vi "Autonomous Independent.vi"   [LabVIEW 2017]
doc: "This VI is called when autonomous begins, and will automatically be terminated when autonomous ends. You can carry out timed or sensor driven robot movement independently without needing to return to the caller."
uses:
  <vilib>/Rock Robotics/WPI/ThirdParty/Sensors/navX/_TypeDefs/FRIC_navX_DeviceNumbersTypeDef.ctl
  <vilib>/Rock Robotics/Network Tables/NT Read String.vi
  Robot Global Data.vi
panel:
  # "Be sure to right-click and choose Data Operations>>Make Current Value default if you want to save the array values with the VI"
types:
  T1 = typedef "FRIC_navX_DeviceNumbersTypeDef.ctl" = enum16{"Dev0", "Dev1", "Dev2", "Dev3"}
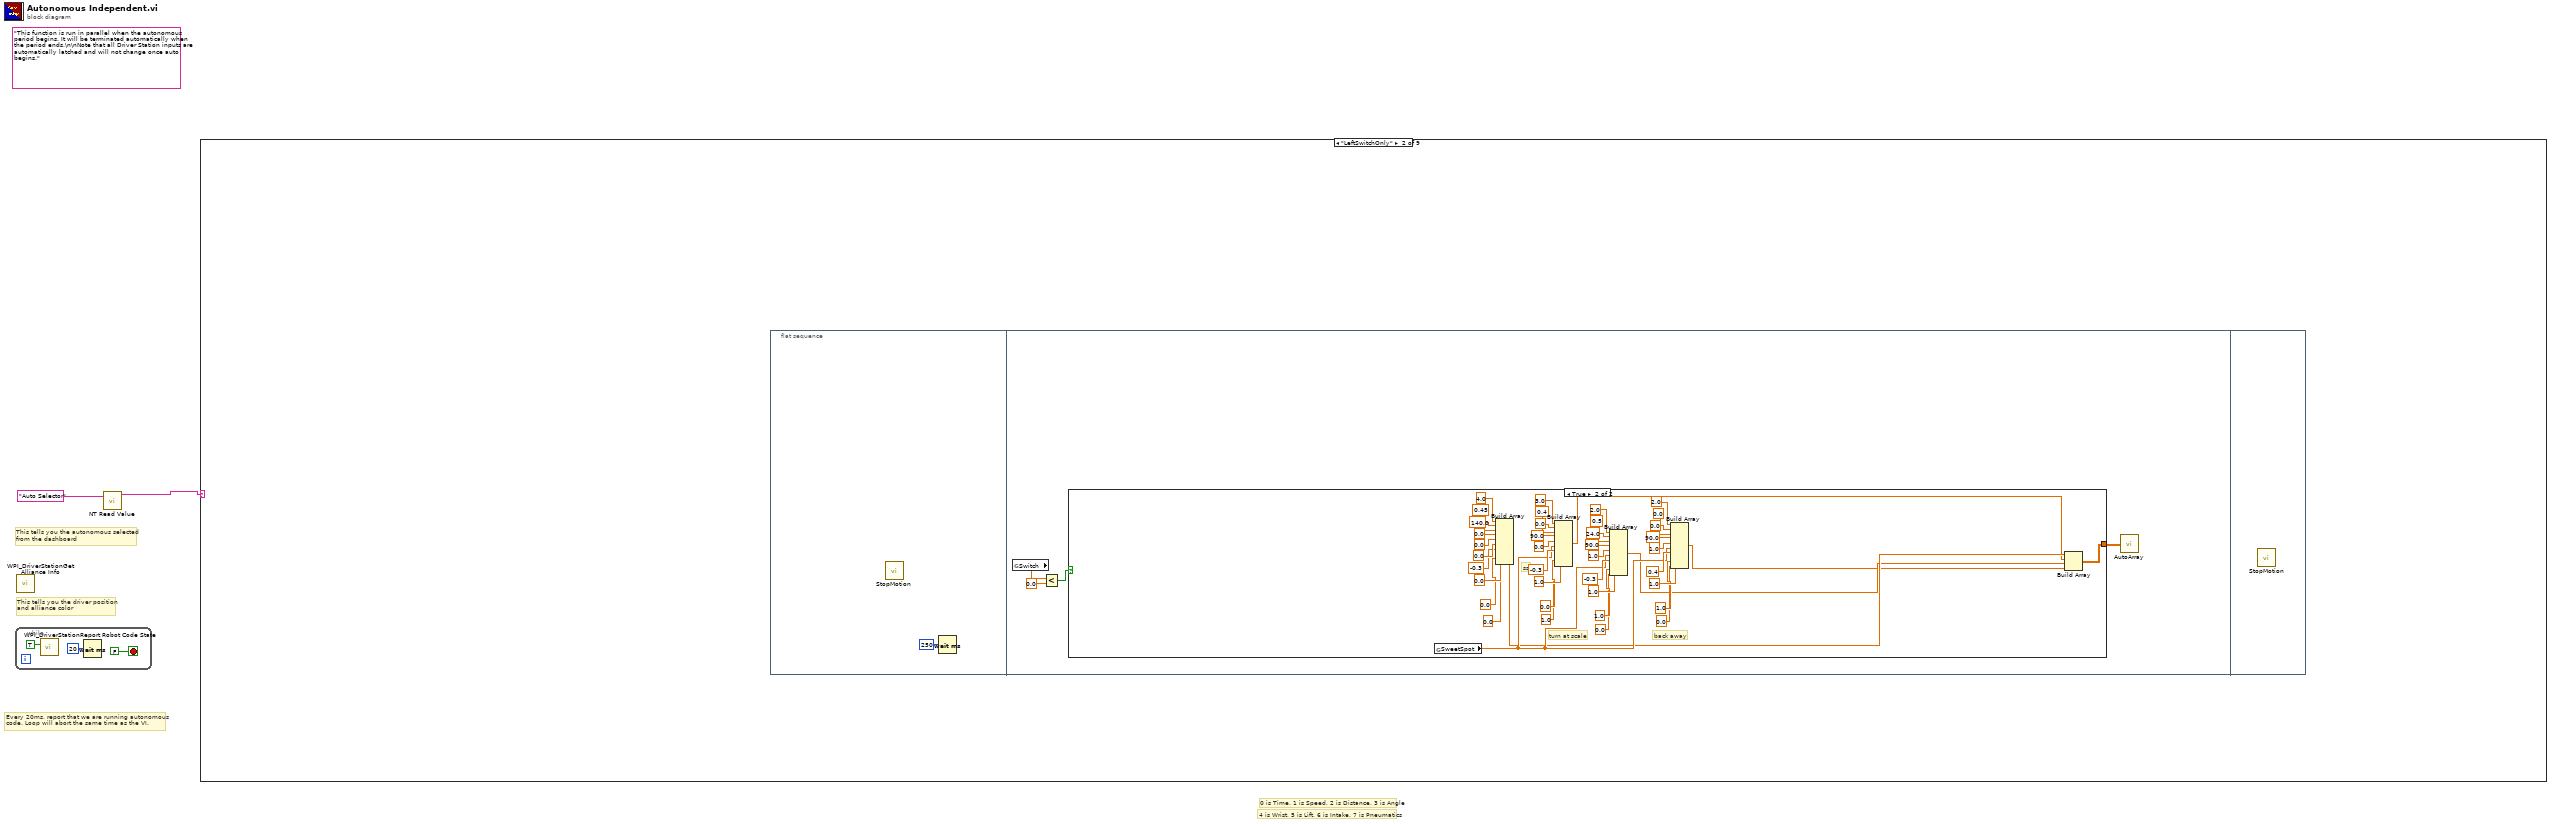
[diagram p0: block diagram]
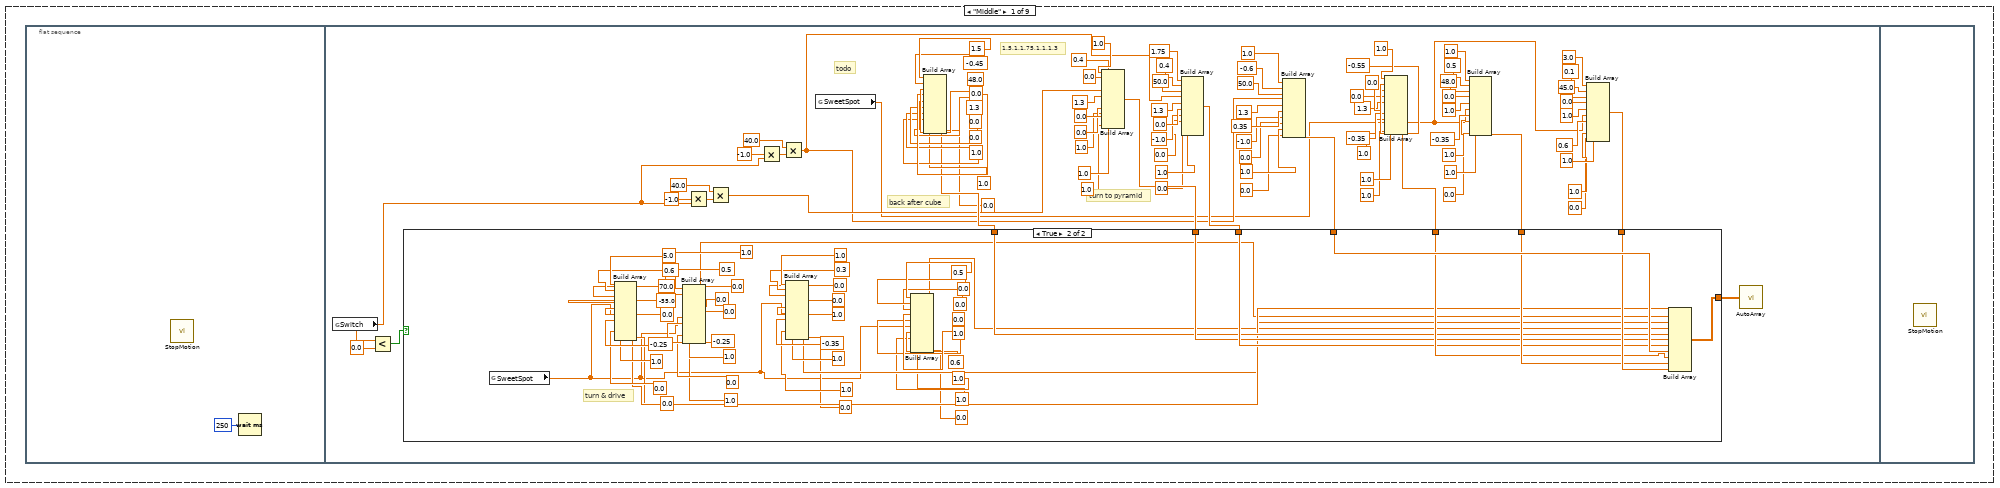
[diagram p2: hidden frame]
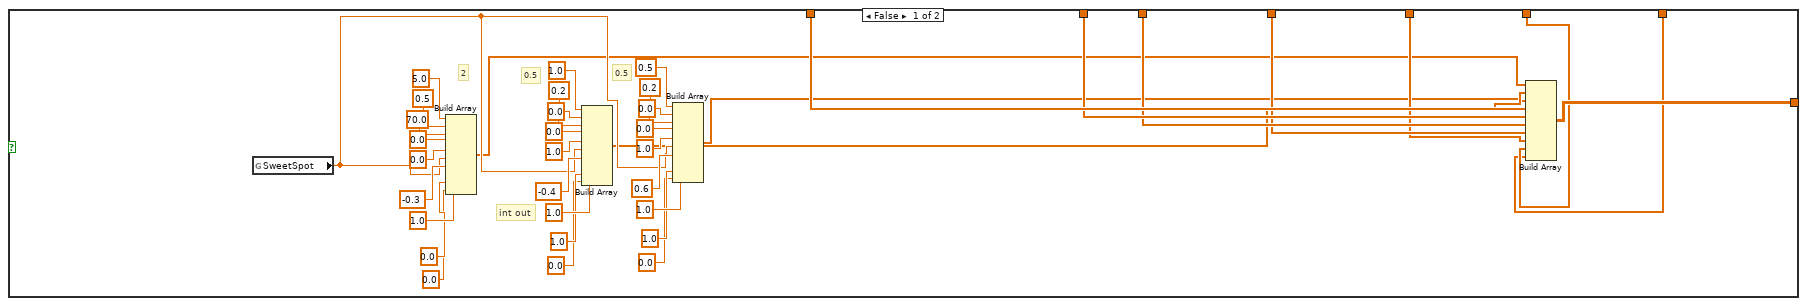
[diagram p3: hidden frame]
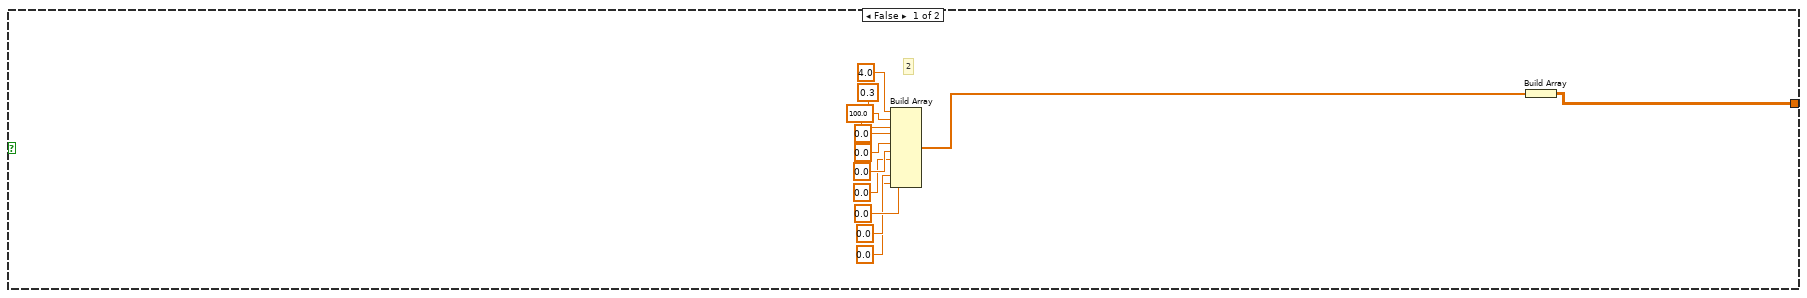
[diagram p4: hidden frame]
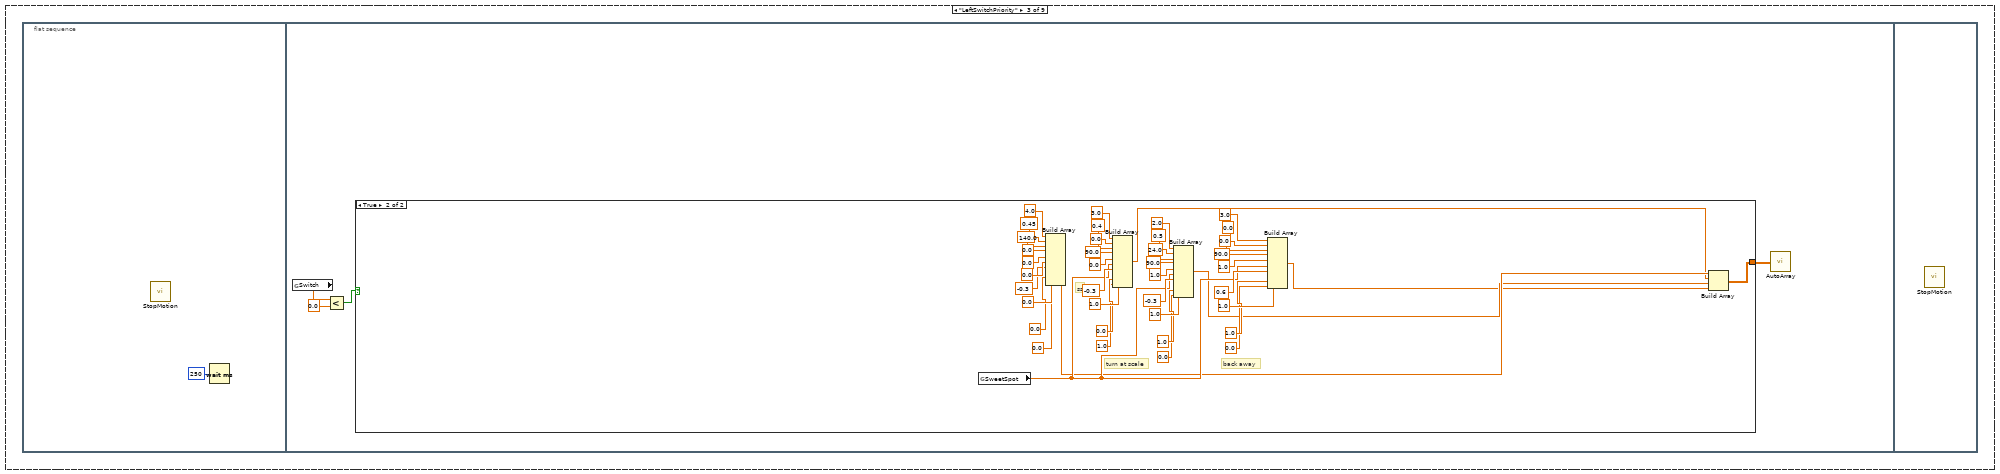
[diagram p5: hidden frame]
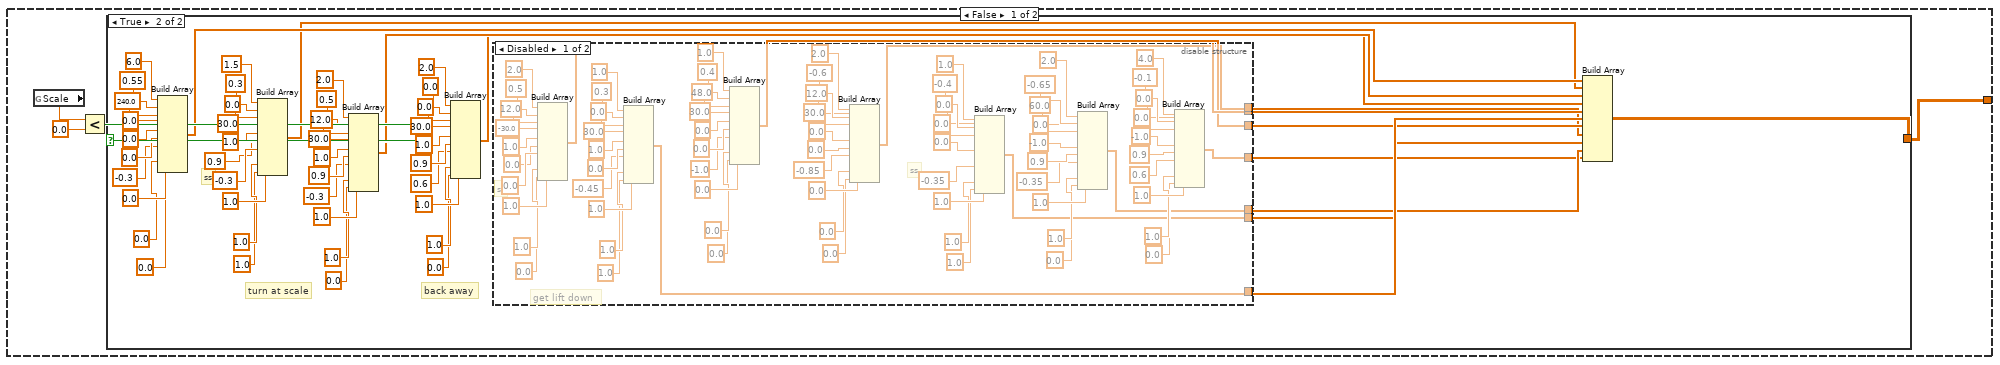
[diagram p6: hidden frame]
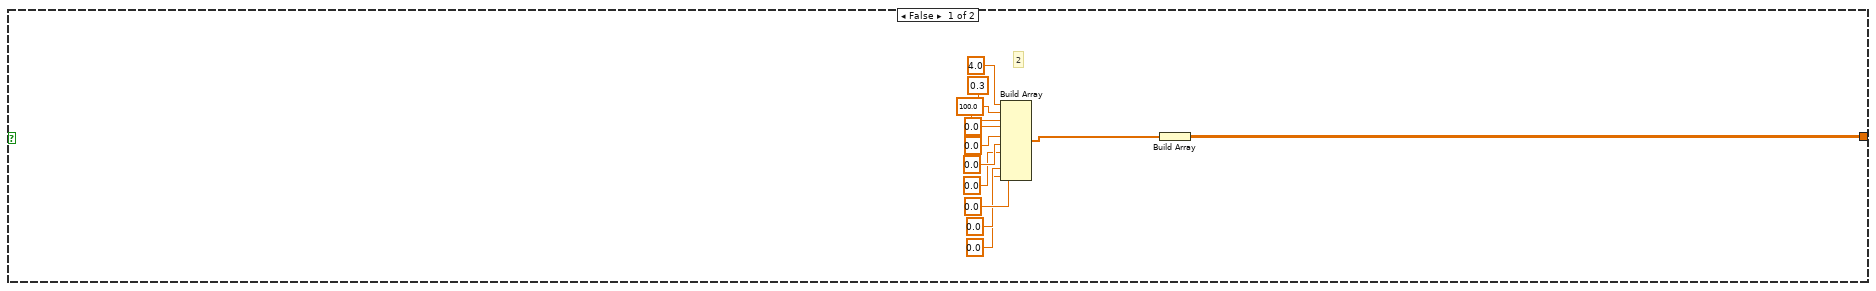
[diagram p7: hidden frame]
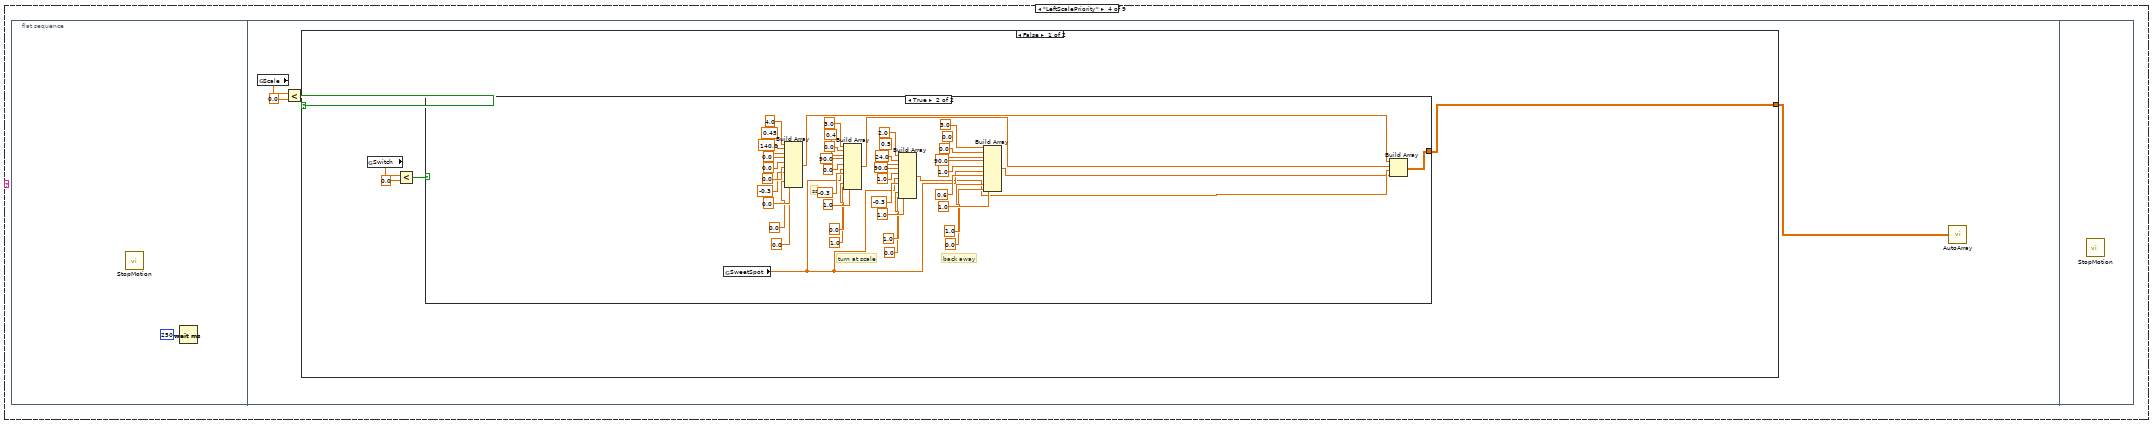
[diagram p9: hidden frame]
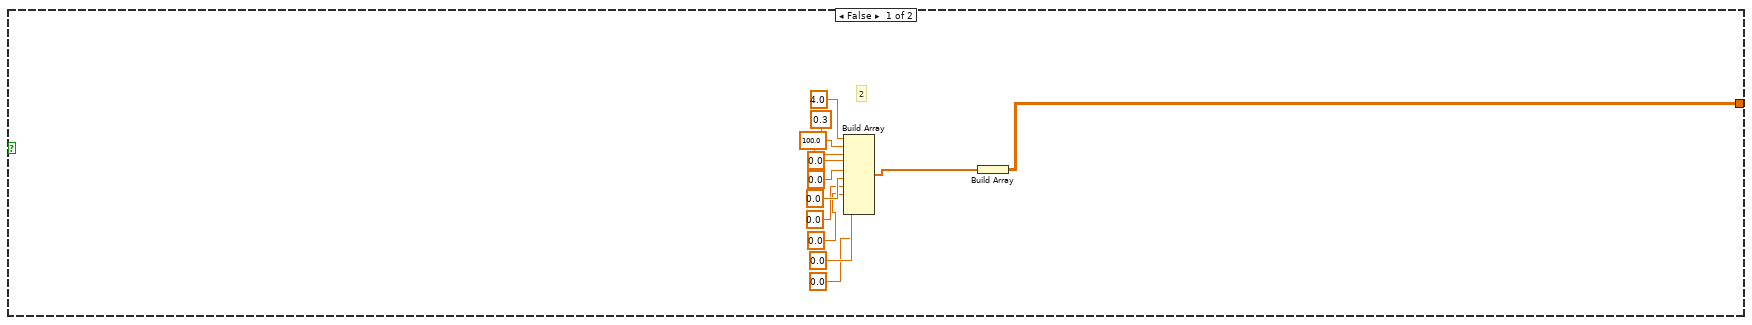
[diagram p10: hidden frame]
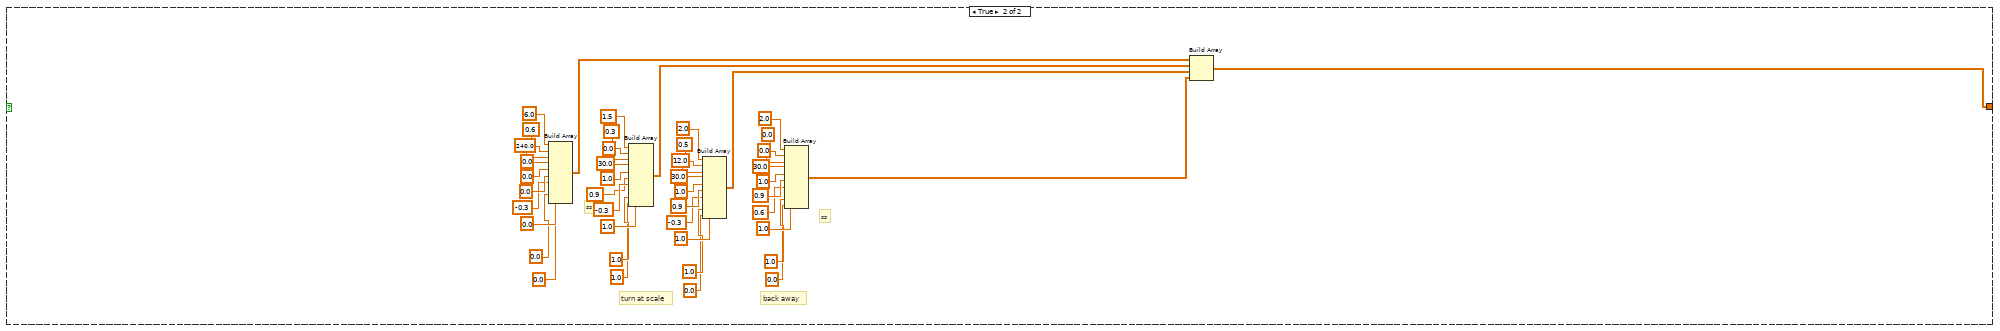
[diagram p11: hidden frame]
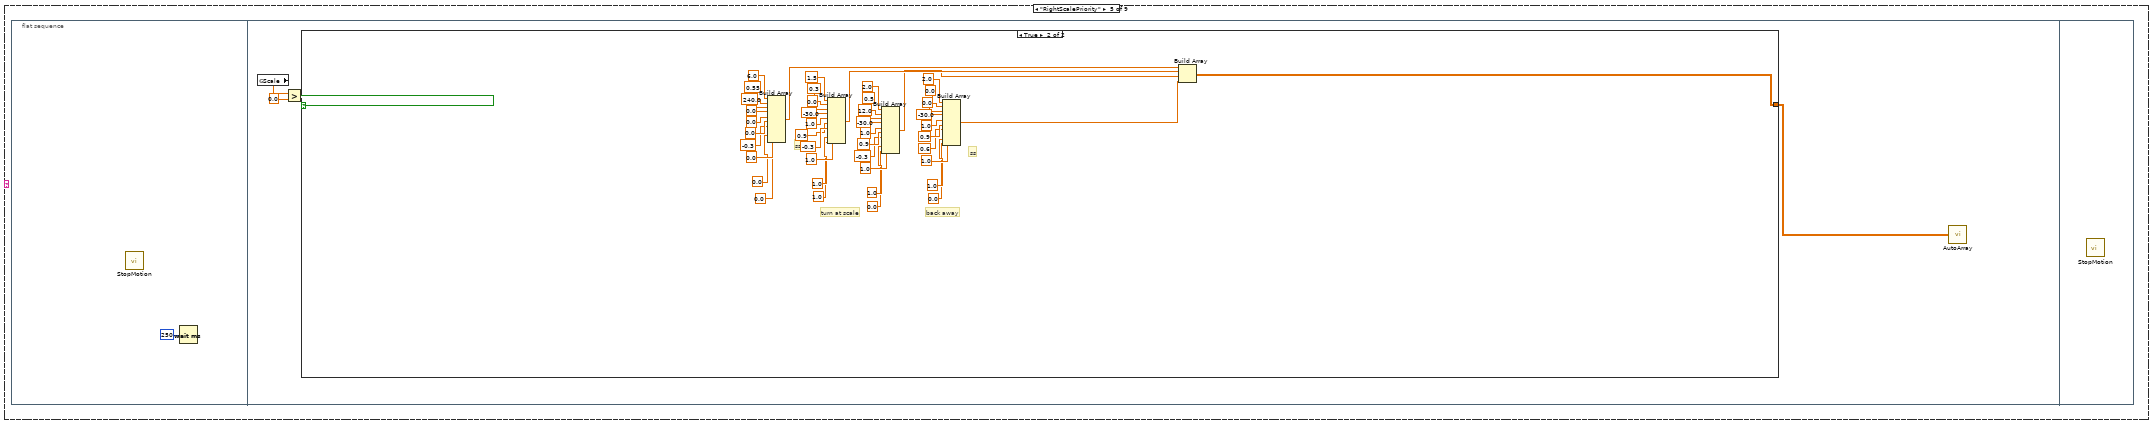
[diagram p12: hidden frame]
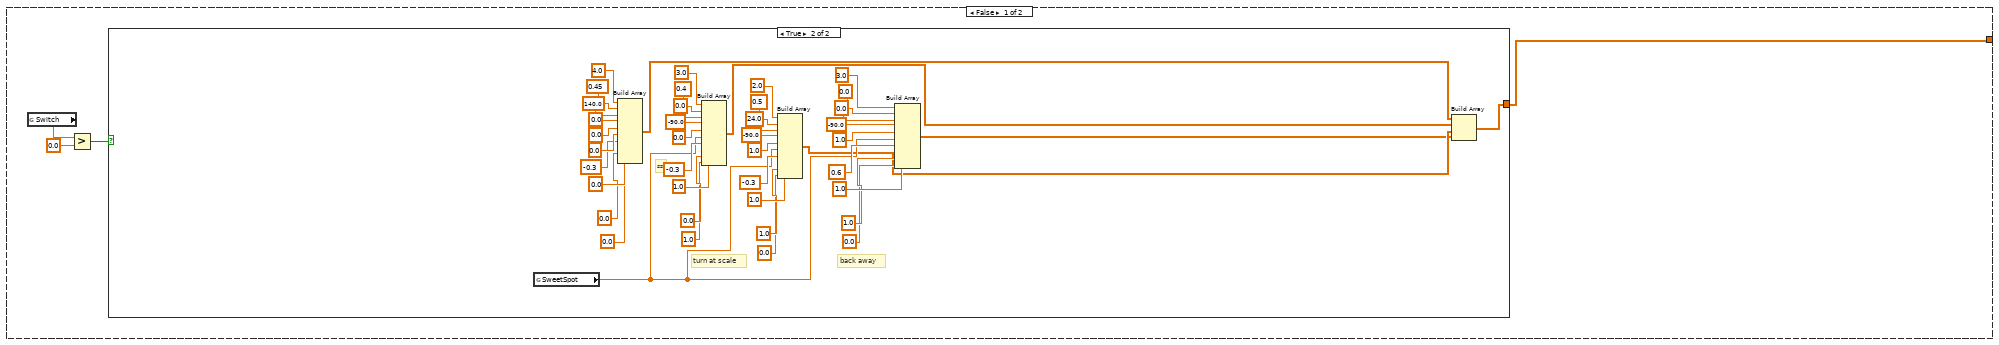
[diagram p13: hidden frame]
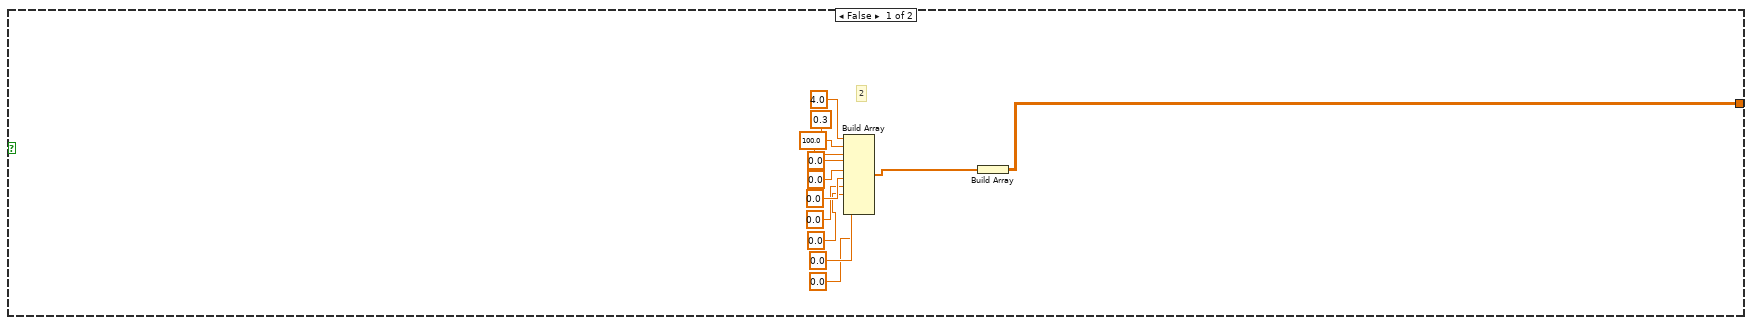
[diagram p14: hidden frame]
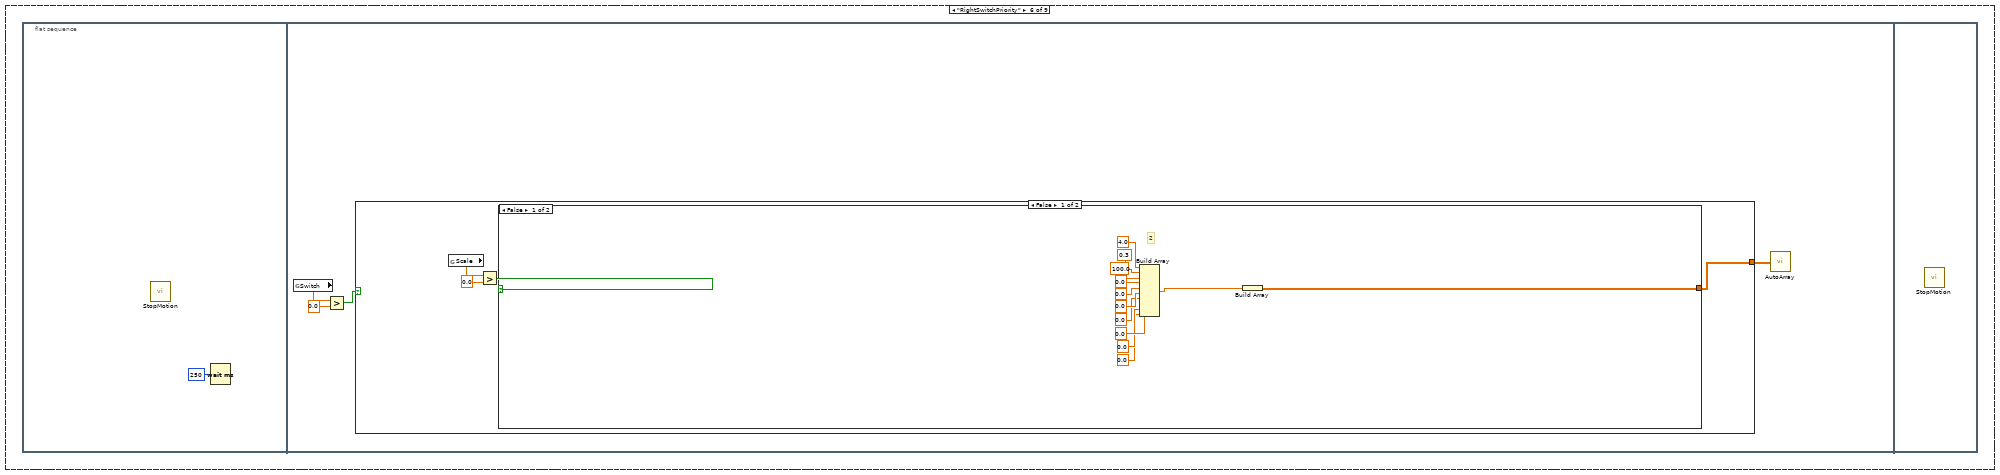
[diagram p15: hidden frame]
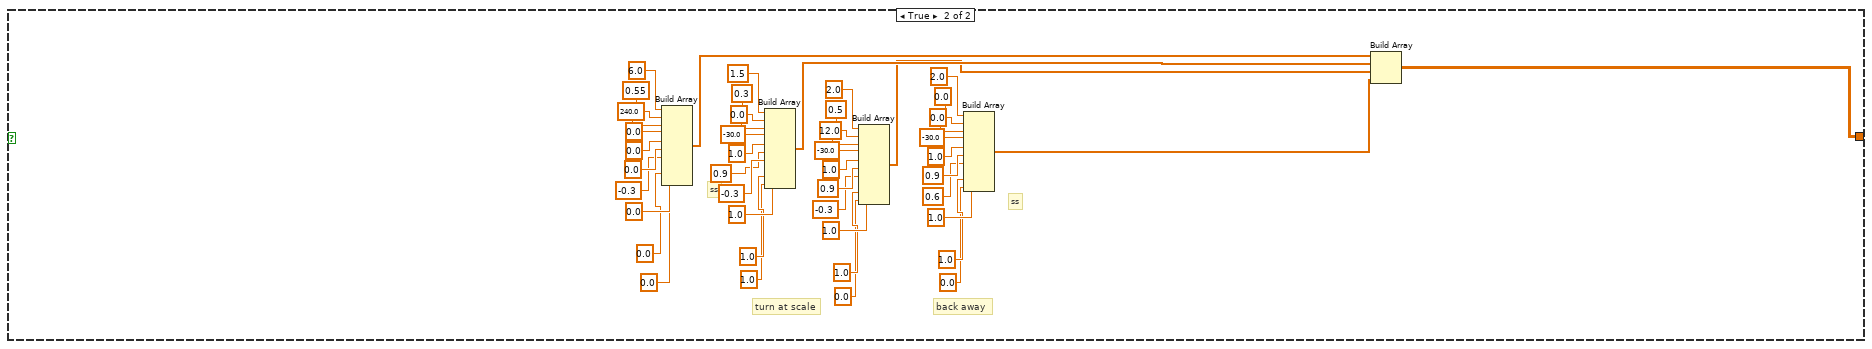
[diagram p16: hidden frame]
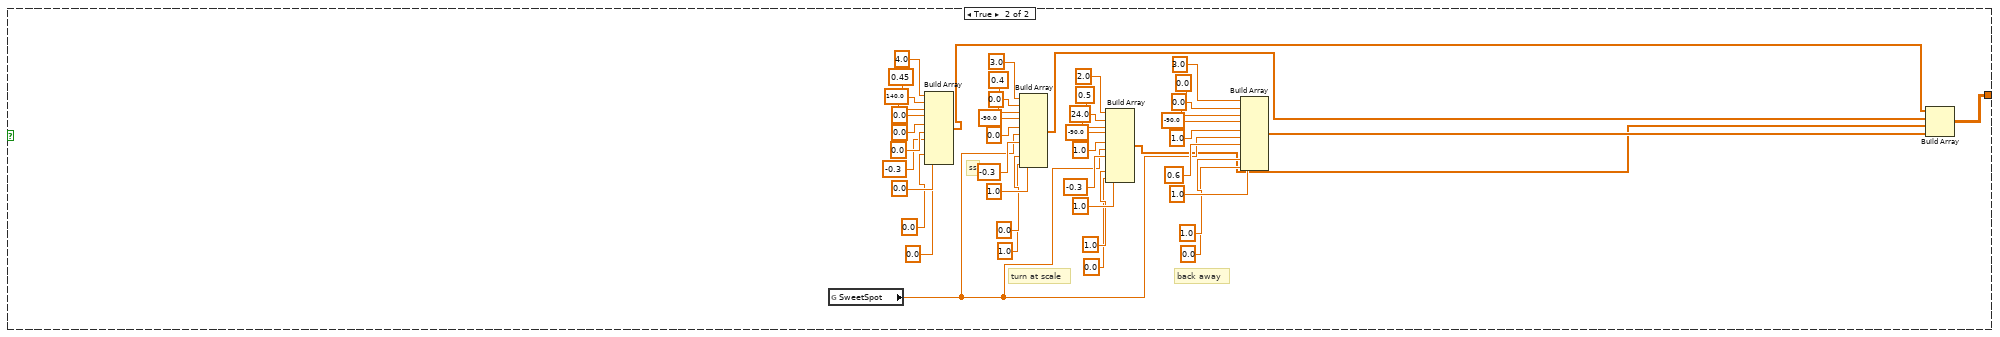
[diagram p17: hidden frame]
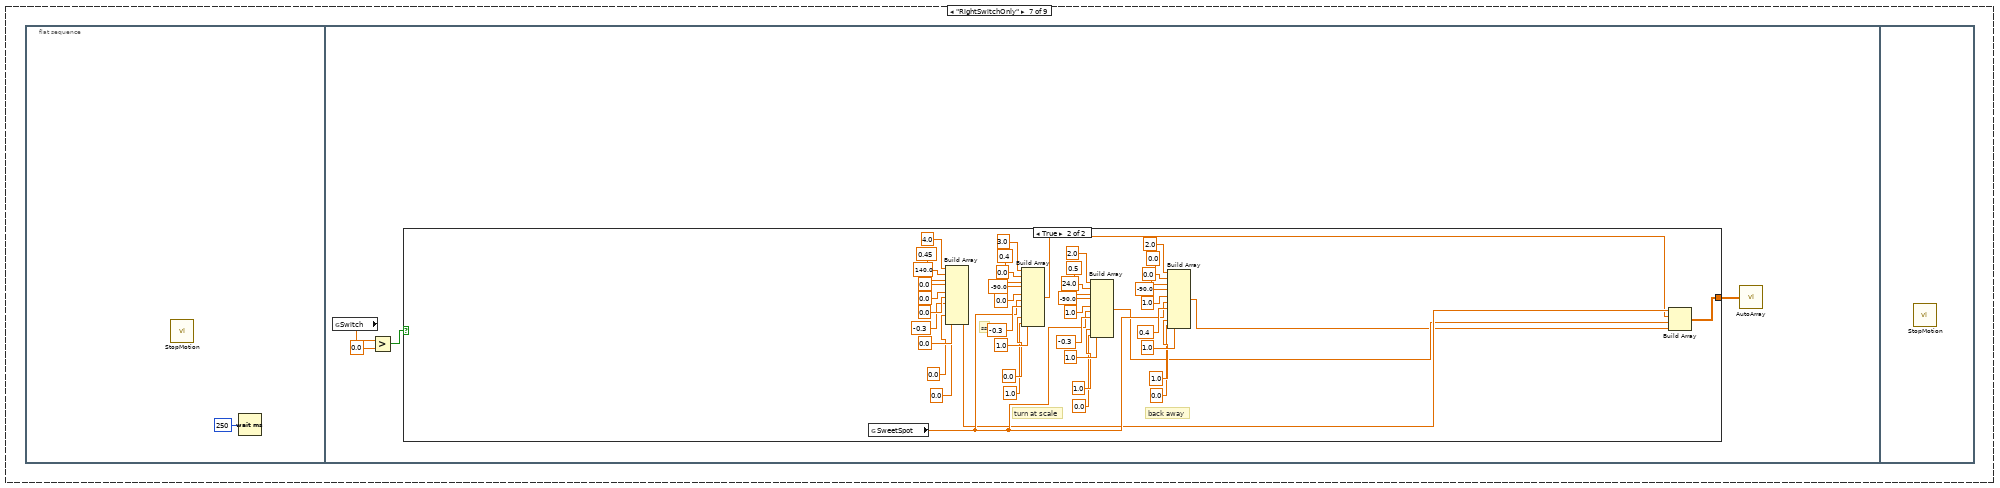
[diagram p18: hidden frame]
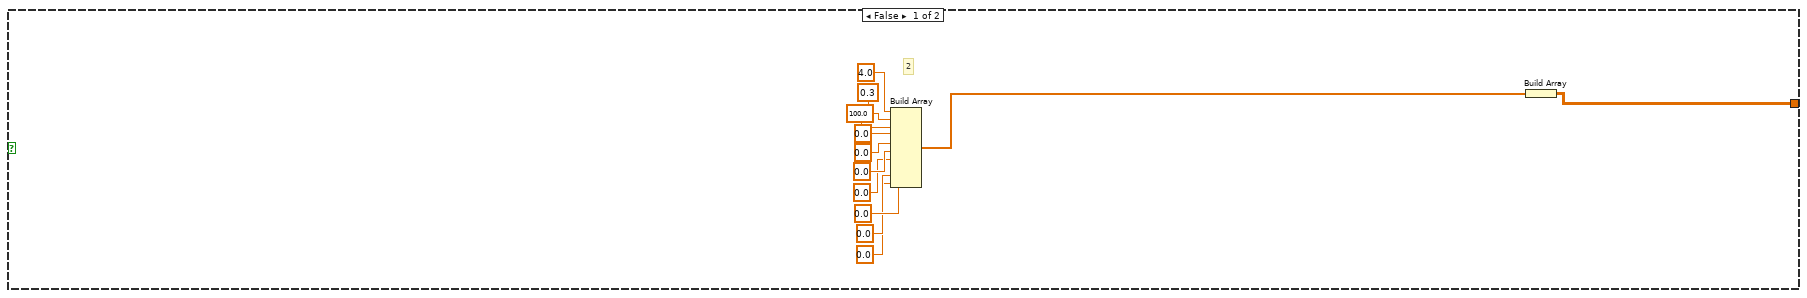
[diagram p19: hidden frame]
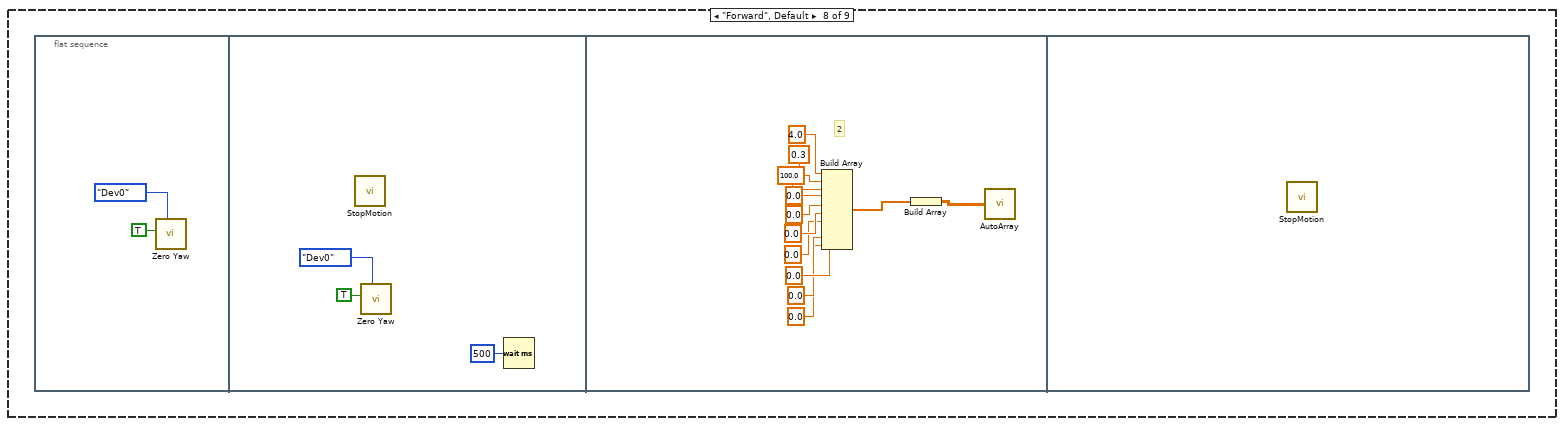
[diagram p20: hidden frame]
diagram:
  (unwired) "This function is run in parallel when the autonomous period begins. It will be terminated automatically when the period ends.\n\nNote that all Driver Station inputs are automatically latched and will not change once auto begins."
  # "4 is Wrist, 5 is Lift, 6 is Intake, 7 is Pneumatics"
  # "0 is Time, 1 is Speed, 2 is Distance, 3 is Angle"
  # "This tells you the autonomous selected\nfrom the dashboard"
  # "Every 20ms, report that we are running autonomous\ncode. Loop will abort the same time as the VI."
  # "This tells you the driver position\nand alliance color"
  n1 = while {
    stop <- FALSE stop-if-true
    n2 = call <vilib>:"WPI_DriverStationReport Robot Code State.vi"("Autonomous"=TRUE) -> ()  [unwired: 10 in, 1 out]
    n3 = Wait (ms)(milliseconds to wait=u32 20) -> ()  [unwired: 1 out]
  }
  n4 = call <vilib>:"WPI_DriverStationGet Alliance Info.vi"() -> ()  [unwired: 12 out]
  n5 = call-poly <vilib>:"NT Read Value.vi"("Name"="Auto Selector") -> ("String"=w1:string)  [unwired: 9 in, 1 out]
  n6 = case shown="\"LeftSwitchOnly\"" w1 {
    frame "Middle" {
      n7 = flat-sequence {
        frame #0 {
          n8 = call "StopMotion.vi"() -> ()  [unwired: 12 in]
          n9 = Wait (ms)(milliseconds to wait=u32 250) -> ()  [unwired: 1 out]
        }
        frame #1 {
          # "1.5,1,1.75,1,1,1,3"
          # "todo"
          # "turn to pyramid"
          # "back after cube"
          n10 = global read "Robot Global Data.vi" "Switch"() -> (w18:dbl)
          n11 = Less?(x=w18, y=0.0) -> (x < y?=w90:bool)
          n12 = Multiply(x=-1.0, y=w18) -> (x*y=w24:dbl)
          n13 = Multiply(x=40.0 ("element"), y=w24) -> (x*y=w17:dbl)
          n14 = Multiply(x=-1.0, y=w18) -> (x*y=w21:dbl)
          n15 = Multiply(x=40.0 ("element"), y=w21) -> (x*y=w16:dbl)
          n16 = global read "Robot Global Data.vi" "SweetSpot"() -> (w7:dbl)
          n17 = Build Array(1.5 ("element"), -0.45 ("element"), 48.0 ("element"), 0.0 ("element"), 1.3 ("element"), 0.0 ("element"), 0.0 ("element"), 1.0 ("element"), 1.0, 0.0 ("element")) -> (w25:dbl[])
          n18 = Build Array(1.0 ("element"), 0.4 ("element"), 0.0 ("element"), w17, 1.3 ("element"), 0.0 ("element"), 0.0 ("element"), 1.0 ("element"), 1.0, 1.0 ("element")) -> (w26:dbl[])
          n19 = Build Array(1.75 ("element"), 0.4 ("element"), 50.0 ("element"), w16, 1.3 ("element"), 0.0 ("element"), -1.0 ("element"), 0.0 ("element"), 1.0 ("element"), 0.0 ("element")) -> (w27:dbl[])
          n20 = Build Array(1.0 ("element"), -0.6 ("element"), 50.0 ("element"), w16, 1.3 ("element"), 0.35 ("element"), -1.0 ("element"), 0.0 ("element"), 1.0 ("element"), 0.0 ("element")) -> (w31:dbl[])
          n21 = Build Array(1.0 ("element"), -0.55 ("element"), 0.0 ("element"), 0.0, 1.3 ("element"), w7, -0.35 ("element"), 1.0 ("element"), 1.0, 1.0 ("element")) -> (w28:dbl[])
          n22 = Build Array(1.0 ("element"), 0.5 ("element"), 48.0 ("element"), 0.0 ("element"), 1.0 ("element"), w7, -0.35 ("element"), 1.0 ("element"), 1.0, 0.0 ("element")) -> (w29:dbl[])
          n23 = Build Array(3.0 ("element"), 0.1 ("element"), 45.0 ("element"), 0.0 ("element"), 1.0 ("element"), w7, 0.6 ("element"), 1.0 ("element"), 1.0, 0.0 ("element")) -> (w30:dbl[])
          n24 = case shown="True" w90 {
            tunnel: w31 -> [w110 w154]
            tunnel: w30 -> [w107 w153]
            tunnel: w29 -> [w108 w152]
            tunnel: w28 -> [w109 w151]
            tunnel: w27 -> [w111 w150]
            tunnel: w26 -> [w112 w149]
            tunnel: w25 -> [w113 w148]
            tunnel: [w114 w144] -> w88
            frame False {
              # "0.5"
              # "int out"
              # "0.5"
              # "2"
              n25 = global read "Robot Global Data.vi" "SweetSpot"() -> (w94:dbl)
              n26 = Build Array(5.0 ("element"), 0.5 ("element"), 70.0 ("element"), 0.0 ("element"), 0.0 ("element"), w94, -0.3 ("element"), 1.0 ("element"), 0.0 ("element"), 0.0 ("element")) -> (w93:dbl[])
              n27 = Build Array(1.0 ("element"), 0.2 ("element"), 0.0 ("element"), 0.0 ("element"), 1.0 ("element"), w94, -0.4 ("element"), 1.0 ("element"), 1.0, 0.0 ("element")) -> (w92:dbl[])
              n28 = Build Array(0.5 ("element"), 0.2 ("element"), 0.0 ("element"), 0.0 ("element"), 1.0 ("element"), w94, 0.6 ("element"), 1.0 ("element"), 1.0, 0.0 ("element")) -> (w91:dbl[])
              n29 = Build Array(w93, w92, w91, w113, w112, w111, w110, w109, w108, w107) -> (w114:dbl[][])
            }
            frame True {
              # "turn & drive"
              n30 = global read "Robot Global Data.vi" "SweetSpot"() -> (w130:dbl)
              n31 = Build Array(5.0 ("element"), 0.6 ("element"), 70.0 ("element"), -55.0 ("AngleSetpoint"), 0.0 ("element"), w130, -0.25 ("element"), 1.0 ("element"), 0.0, 0.0 ("element")) -> (w147:dbl[])
              n32 = Build Array(1.0 ("element"), 0.5 ("element"), 0.0 ("element"), 0.0, 0.0 ("element"), w130, -0.25 ("element"), 1.0 ("element"), 0.0, 1.0 ("element")) -> (w146:dbl[])
              n33 = Build Array(1.0 ("element"), 0.3 ("element"), 0.0 ("element"), 0.0 ("element"), 1.0 ("element"), w130, -0.35 ("element"), 1.0 ("element"), 1.0, 0.0 ("element")) -> (w145:dbl[])
              n34 = Build Array(0.5 ("element"), 0.0 ("element"), 0.0 ("element"), 0.0 ("element"), 1.0 ("element"), w130, 0.6 ("element"), 1.0 ("element"), 1.0, 0.0 ("element")) -> (w135:dbl[])
              n35 = Build Array(w147, w146, w145, w135, w148, w149, w150, w154, w151, w152, w153) -> (w144:dbl[][])
            }
          }
          n36 = call "AutoArray.vi"("Array"=w88) -> ()
        }
        frame #2 {
          n37 = call "StopMotion.vi"() -> ()  [unwired: 12 in]
        }
      }
    }
    frame "LeftSwitchOnly" {
      n38 = flat-sequence {
        frame #0 {
          n39 = call "StopMotion.vi"() -> ()  [unwired: 12 in]
          n40 = Wait (ms)(milliseconds to wait=u32 250) -> ()  [unwired: 1 out]
        }
        frame #1 {
          n41 = global read "Robot Global Data.vi" "Switch"() -> (w180:dbl)
          n42 = Less?(x=w180, y=0.0) -> (x < y?=w183:bool)
          n43 = case shown="True" w183 {
            tunnel: [w184 w196] -> w181
            frame False {
              # "2"
              n44 = Build Array(4.0 ("element"), 0.3 ("element"), 100.0 ("element"), 0.0 ("element"), 0.0 ("element"), 0.0 ("element"), 0.0 ("element"), 0.0 ("element"), 0.0 ("element"), 0.0 ("element")) -> (w185:dbl[])
              n45 = Build Array(w185) -> (w184:dbl[][])
            }
            frame True {
              # "ss"
              # "back away"
              # "turn at scale"
              n46 = global read "Robot Global Data.vi" "SweetSpot"() -> (w201:dbl)
              n47 = Build Array(4.0 ("element"), 0.45 ("element"), 140.0 ("element"), 0.0 ("element"), 0.0 ("element"), 0.0 ("element"), -0.3 ("element"), 0.0 ("element"), 0.0, 0.0 ("element")) -> (w200:dbl[])
              n48 = Build Array(3.0 ("element"), 0.4 ("element"), 0.0 ("element"), 90.0 ("element"), 0.0 ("element"), w201, -0.3 ("element"), 1.0 ("element"), 0.0, 1.0 ("element")) -> (w199:dbl[])
              n49 = Build Array(2.0 ("element"), 0.5 ("element"), 24.0 ("element"), 90.0 ("element"), 1.0 ("element"), w201, -0.3 ("element"), 1.0 ("element"), 1.0, 0.0 ("element")) -> (w198:dbl[])
              n50 = Build Array(2.0 ("element"), 0.0 ("element"), 0.0 ("element"), 90.0 ("element"), 1.0 ("element"), w201, 0.4 ("element"), 1.0 ("element"), 1.0, 0.0 ("element")) -> (w197:dbl[])
              n51 = Build Array(w200, w199, w198, w197) -> (w196:dbl[][])
            }
          }
          n52 = call "AutoArray.vi"("Array"=w181) -> ()
        }
        frame #2 {
          n53 = call "StopMotion.vi"() -> ()  [unwired: 12 in]
        }
      }
    }
    frame "LeftSwitchPriority" {
      n54 = flat-sequence {
        frame #0 {
          n55 = call "StopMotion.vi"() -> ()  [unwired: 12 in]
          n56 = Wait (ms)(milliseconds to wait=u32 250) -> ()  [unwired: 1 out]
        }
        frame #1 {
          n57 = global read "Robot Global Data.vi" "Switch"() -> (w241:dbl)
          n58 = Less?(x=w241, y=0.0) -> (x < y?=w243:bool)
          n59 = case shown="True" w243 {
            tunnel: [w244 w388] -> w240
            frame False {
              n60 = global read "Robot Global Data.vi" "Scale"() -> (w246:dbl)
              n61 = Less?(x=w246, y=0.0) -> (x < y?=w245:bool)
              n62 = case shown="True" w245 {
                tunnel: [w248 w272] -> w244
                frame False {
                  # "2"
                  n63 = Build Array(4.0 ("element"), 0.3 ("element"), 100.0 ("element"), 0.0 ("element"), 0.0 ("element"), 0.0 ("element"), 0.0 ("element"), 0.0 ("element"), 0.0 ("element"), 0.0 ("element")) -> (w249:dbl[])
                  n64 = Build Array(w249) -> (w248:dbl[][])
                }
                frame True {
                  # "ss"
                  # "back away"
                  # "turn at scale"
                  n65 = Build Array(6.0 ("element"), 0.55 ("element"), 240.0 ("element"), 0.0 ("element"), 0.0 ("element"), 0.0 ("element"), -0.3 ("element"), 0.0 ("element"), 0.0, 0.0 ("element")) -> (w271:dbl[])
                  n66 = Build Array(1.5 ("element"), 0.3 ("element"), 0.0 ("element"), 30.0 ("element"), 1.0 ("element"), 0.9, -0.3 ("element"), 1.0 ("element"), 1.0, 1.0 ("element")) -> (w270:dbl[])
                  n67 = Build Array(2.0 ("element"), 0.5 ("element"), 12.0 ("element"), 30.0 ("element"), 1.0 ("element"), 0.9 ("element"), -0.3 ("element"), 1.0 ("element"), 1.0, 0.0 ("element")) -> (w269:dbl[])
                  n68 = Build Array(2.0 ("element"), 0.0 ("element"), 0.0 ("element"), 30.0 ("element"), 1.0 ("element"), 0.9 ("element"), 0.6 ("element"), 1.0 ("element"), 1.0, 0.0 ("element")) -> (w268:dbl[])
                  n69 = disable-structure shown="Disabled" {
                    disable-tunnel: [w319 _] -> w267
                    disable-tunnel: [w318 _] -> w266
                    disable-tunnel: [w317 _] -> w265
                    disable-tunnel: [w316 _] -> w264
                    disable-tunnel: [w315 _] -> w263
                    disable-tunnel: [w314 _] -> w262
                    disable-tunnel: [w313 _] -> w261
                    frame Disabled {
                      # "ss"
                      # "ss"
                      # "get lift down"
                      n70 = Build Array(2.0 ("element"), 0.5 ("element"), 12.0 ("element"), -30.0 ("element"), 1.0 ("element"), 0.0 ("element"), 0.0 ("element"), 1.0 ("element"), 1.0, 0.0 ("element")) -> (w319:dbl[])
                      n71 = Build Array(1.0 ("element"), 0.3 ("element"), 0.0 ("element"), 30.0 ("element"), 1.0 ("element"), 0.0 ("element"), -0.45 ("element"), 1.0 ("element"), 1.0, 1.0 ("element")) -> (w318:dbl[])
                      n72 = Build Array(1.0 ("element"), 0.4 ("element"), 48.0 ("element"), 30.0 ("element"), 0.0 ("element"), 0.0 ("element"), -1.0 ("element"), 0.0 ("element"), 0.0, 0.0 ("element")) -> (w317:dbl[])
                      n73 = Build Array(2.0 ("element"), -0.6 ("element"), 12.0 ("element"), 30.0 ("element"), 0.0 ("element"), 0.0 ("element"), -0.85 ("element"), 0.0 ("element"), 0.0, 0.0 ("element")) -> (w316:dbl[])
                      n74 = Build Array(1.0 ("element"), -0.4 ("element"), 0.0 ("element"), 0.0 ("element"), 0.0 ("element"), -0.35 ("element"), 1.0 ("element"), 1.0, 1.0 ("element")) -> (w315:dbl[])  [unwired: 1 in]
                      n75 = Build Array(2.0 ("element"), -0.65 ("element"), 60.0 ("element"), 0.0 ("element"), -1.0 ("element"), 0.9 ("element"), -0.35 ("element"), 1.0 ("element"), 1.0, 0.0 ("element")) -> (w314:dbl[])
                      n76 = Build Array(4.0 ("element"), -0.1 ("element"), 0.0 ("element"), 0.0 ("element"), -1.0 ("element"), 0.9 ("element"), 0.6 ("element"), 1.0 ("element"), 1.0, 0.0 ("element")) -> (w313:dbl[])
                    }
                    frame Enabled {
                    }
                  }
                  n77 = Build Array(w271, w270, w269, w268, w267, w266, w265, w264, w263, w262, w261) -> (w272:dbl[][])
                }
              }
            }
            frame True {
              # "ss"
              # "back away"
              # "turn at scale"
              n78 = global read "Robot Global Data.vi" "SweetSpot"() -> (w393:dbl)
              n79 = Build Array(4.0 ("element"), 0.45 ("element"), 140.0 ("element"), 0.0 ("element"), 0.0 ("element"), 0.0 ("element"), -0.3 ("element"), 0.0 ("element"), 0.0, 0.0 ("element")) -> (w392:dbl[])
              n80 = Build Array(3.0 ("element"), 0.4 ("element"), 0.0 ("element"), 90.0 ("element"), 0.0 ("element"), w393, -0.3 ("element"), 1.0 ("element"), 0.0, 1.0 ("element")) -> (w391:dbl[])
              n81 = Build Array(2.0 ("element"), 0.5 ("element"), 24.0 ("element"), 90.0 ("element"), 1.0 ("element"), w393, -0.3 ("element"), 1.0 ("element"), 1.0, 0.0 ("element")) -> (w390:dbl[])
              n82 = Build Array(3.0 ("element"), 0.0 ("element"), 0.0 ("element"), 90.0 ("element"), 1.0 ("element"), w393, 0.6 ("element"), 1.0 ("element"), 1.0, 0.0 ("element")) -> (w389:dbl[])
              n83 = Build Array(w392, w391, w390, w389) -> (w388:dbl[][])
            }
          }
          n84 = call "AutoArray.vi"("Array"=w240) -> ()
        }
        frame #2 {
          n85 = call "StopMotion.vi"() -> ()  [unwired: 12 in]
        }
      }
    }
    frame "LeftScalePriority" {
      n86 = flat-sequence {
        frame #0 {
          n87 = call "StopMotion.vi"() -> ()  [unwired: 12 in]
          n88 = Wait (ms)(milliseconds to wait=u32 250) -> ()  [unwired: 1 out]
        }
        frame #1 {
          n89 = global read "Robot Global Data.vi" "Scale"() -> (w434:dbl)
          n90 = Less?(x=w434, y=0.0) -> (x < y?=w433:bool)
          n91 = case shown="False" w433 {
            tunnel: [w437 w495] -> w432
            frame False {
              n92 = global read "Robot Global Data.vi" "Switch"() -> (w438:dbl)
              n93 = Less?(x=w438, y=0.0) -> (x < y?=w436:bool)
              n94 = case shown="True" w436 {
                tunnel: [w440 w494] -> w437
                frame False {
                  # "2"
                  n95 = Build Array(4.0 ("element"), 0.3 ("element"), 100.0 ("element"), 0.0 ("element"), 0.0 ("element"), 0.0 ("element"), 0.0 ("element"), 0.0 ("element"), 0.0 ("element"), 0.0 ("element")) -> (w441:dbl[])
                  n96 = Build Array(w441) -> (w440:dbl[][])
                }
                frame True {
                  # "ss"
                  # "back away"
                  # "turn at scale"
                  n97 = global read "Robot Global Data.vi" "SweetSpot"() -> (w456:dbl)
                  n98 = Build Array(4.0 ("element"), 0.45 ("element"), 140.0 ("element"), 0.0 ("element"), 0.0 ("element"), 0.0 ("element"), -0.3 ("element"), 0.0 ("element"), 0.0, 0.0 ("element")) -> (w455:dbl[])
                  n99 = Build Array(3.0 ("element"), 0.4 ("element"), 0.0 ("element"), 90.0 ("element"), 0.0 ("element"), w456, -0.3 ("element"), 1.0 ("element"), 0.0, 1.0 ("element")) -> (w454:dbl[])
                  n100 = Build Array(2.0 ("element"), 0.5 ("element"), 24.0 ("element"), 90.0 ("element"), 1.0 ("element"), w456, -0.3 ("element"), 1.0 ("element"), 1.0, 0.0 ("element")) -> (w453:dbl[])
                  n101 = Build Array(3.0 ("element"), 0.0 ("element"), 0.0 ("element"), 90.0 ("element"), 1.0 ("element"), w456, 0.6 ("element"), 1.0 ("element"), 1.0, 0.0 ("element")) -> (w452:dbl[])
                  n102 = Build Array(w455, w454, w453, w452) -> (w494:dbl[][])
                }
              }
            }
            frame True {
              # "ss"
              # "ss"
              # "back away"
              # "turn at scale"
              n103 = Build Array(6.0 ("element"), 0.6 ("element"), 240.0 ("element"), 0.0 ("element"), 0.0 ("element"), 0.0 ("element"), -0.3 ("element"), 0.0 ("element"), 0.0, 0.0 ("element")) -> (w499:dbl[])
              n104 = Build Array(1.5 ("element"), 0.3 ("element"), 0.0 ("element"), 30.0 ("element"), 1.0 ("element"), 0.9, -0.3 ("element"), 1.0 ("element"), 1.0, 1.0 ("element")) -> (w498:dbl[])
              n105 = Build Array(2.0 ("element"), 0.5 ("element"), 12.0 ("element"), 30.0 ("element"), 1.0 ("element"), 0.9 ("element"), -0.3 ("element"), 1.0 ("element"), 1.0, 0.0 ("element")) -> (w497:dbl[])
              n106 = Build Array(2.0 ("element"), 0.0 ("element"), 0.0 ("element"), 30.0 ("element"), 1.0 ("element"), 0.9 ("element"), 0.6 ("element"), 1.0 ("element"), 1.0, 0.0 ("element")) -> (w496:dbl[])
              n107 = Build Array(w499, w498, w497, w496) -> (w495:dbl[][])
            }
          }
          n108 = call "AutoArray.vi"("Array"=w432) -> ()
        }
        frame #2 {
          n109 = call "StopMotion.vi"() -> ()  [unwired: 12 in]
        }
      }
    }
    frame "RightScalePriority" {
      n110 = flat-sequence {
        frame #0 {
          n111 = call "StopMotion.vi"() -> ()  [unwired: 12 in]
          n112 = Wait (ms)(milliseconds to wait=u32 250) -> ()  [unwired: 1 out]
        }
        frame #1 {
          n113 = global read "Robot Global Data.vi" "Scale"() -> (w543:dbl)
          n114 = Greater?(x=w543, y=0.0) -> (0:w542:bool)
          n115 = case shown="True" w542 {
            tunnel: [w546 w604] -> w541
            frame False {
              n116 = global read "Robot Global Data.vi" "Switch"() -> (w547:dbl)
              n117 = Greater?(x=w547, y=0.0) -> (0:w545:bool)
              n118 = case shown="True" w545 {
                tunnel: [w549 w603] -> w546
                frame False {
                  # "2"
                  n119 = Build Array(4.0 ("element"), 0.3 ("element"), 100.0 ("element"), 0.0 ("element"), 0.0 ("element"), 0.0 ("element"), 0.0 ("element"), 0.0 ("element"), 0.0 ("element"), 0.0 ("element")) -> (w550:dbl[])
                  n120 = Build Array(w550) -> (w549:dbl[][])
                }
                frame True {
                  # "ss"
                  # "back away"
                  # "turn at scale"
                  n121 = global read "Robot Global Data.vi" "SweetSpot"() -> (w567:dbl)
                  n122 = Build Array(4.0 ("element"), 0.45 ("element"), 140.0 ("element"), 0.0 ("element"), 0.0 ("element"), 0.0 ("element"), -0.3 ("element"), 0.0 ("element"), 0.0, 0.0 ("element")) -> (w566:dbl[])
                  n123 = Build Array(3.0 ("element"), 0.4 ("element"), 0.0 ("element"), -90.0 ("element"), 0.0 ("element"), w567, -0.3 ("element"), 1.0 ("element"), 0.0, 1.0 ("element")) -> (w565:dbl[])
                  n124 = Build Array(2.0 ("element"), 0.5 ("element"), 24.0 ("element"), -90.0 ("element"), 1.0 ("element"), w567, -0.3 ("element"), 1.0 ("element"), 1.0, 0.0 ("element")) -> (w564:dbl[])
                  n125 = Build Array(3.0 ("element"), 0.0 ("element"), 0.0 ("element"), -90.0 ("element"), 1.0 ("element"), w567, 0.6 ("element"), 1.0 ("element"), 1.0, 0.0 ("element")) -> (w563:dbl[])
                  n126 = Build Array(w566, w565, w564, w563) -> (w603:dbl[][])
                }
              }
            }
            frame True {
              # "ss"
              # "ss"
              # "back away"
              # "turn at scale"
              n127 = Build Array(6.0 ("element"), 0.55 ("element"), 240.0 ("element"), 0.0 ("element"), 0.0 ("element"), 0.0 ("element"), -0.3 ("element"), 0.0 ("element"), 0.0, 0.0 ("element")) -> (w608:dbl[])
              n128 = Build Array(1.5 ("element"), 0.3 ("element"), 0.0 ("element"), -30.0 ("element"), 1.0 ("element"), 0.9, -0.3 ("element"), 1.0 ("element"), 1.0, 1.0 ("element")) -> (w607:dbl[])
              n129 = Build Array(2.0 ("element"), 0.5 ("element"), 12.0 ("element"), -30.0 ("element"), 1.0 ("element"), 0.9 ("element"), -0.3 ("element"), 1.0 ("element"), 1.0, 0.0 ("element")) -> (w606:dbl[])
              n130 = Build Array(2.0 ("element"), 0.0 ("element"), 0.0 ("element"), -30.0 ("element"), 1.0 ("element"), 0.9 ("element"), 0.6 ("element"), 1.0 ("element"), 1.0, 0.0 ("element")) -> (w605:dbl[])
              n131 = Build Array(w608, w607, w606, w605) -> (w604:dbl[][])
            }
          }
          n132 = call "AutoArray.vi"("Array"=w541) -> ()
        }
        frame #2 {
          n133 = call "StopMotion.vi"() -> ()  [unwired: 12 in]
        }
      }
    }
    frame "RightSwitchPriority" {
      n134 = flat-sequence {
        frame #0 {
          n135 = call "StopMotion.vi"() -> ()  [unwired: 12 in]
          n136 = Wait (ms)(milliseconds to wait=u32 250) -> ()  [unwired: 1 out]
        }
        frame #1 {
          n137 = global read "Robot Global Data.vi" "Switch"() -> (w651:dbl)
          n138 = Greater?(x=w651, y=0.0) -> (0:w653:bool)
          n139 = case shown="False" w653 {
            tunnel: [w654 w757] -> w650
            frame False {
              n140 = global read "Robot Global Data.vi" "Scale"() -> (w656:dbl)
              n141 = Greater?(x=w656, y=0.0) -> (0:w655:bool)
              n142 = case shown="False" w655 {
                tunnel: [w658 w670] -> w654
                frame False {
                  # "2"
                  n143 = Build Array(4.0 ("element"), 0.3 ("element"), 100.0 ("element"), 0.0 ("element"), 0.0 ("element"), 0.0 ("element"), 0.0 ("element"), 0.0 ("element"), 0.0 ("element"), 0.0 ("element")) -> (w659:dbl[])
                  n144 = Build Array(w659) -> (w658:dbl[][])
                }
                frame True {
                  # "ss"
                  # "ss"
                  # "back away"
                  # "turn at scale"
                  n145 = Build Array(6.0 ("element"), 0.55 ("element"), 240.0 ("element"), 0.0 ("element"), 0.0 ("element"), 0.0 ("element"), -0.3 ("element"), 0.0 ("element"), 0.0, 0.0 ("element")) -> (w674:dbl[])
                  n146 = Build Array(1.5 ("element"), 0.3 ("element"), 0.0 ("element"), -30.0 ("element"), 1.0 ("element"), 0.9, -0.3 ("element"), 1.0 ("element"), 1.0, 1.0 ("element")) -> (w673:dbl[])
                  n147 = Build Array(2.0 ("element"), 0.5 ("element"), 12.0 ("element"), -30.0 ("element"), 1.0 ("element"), 0.9 ("element"), -0.3 ("element"), 1.0 ("element"), 1.0, 0.0 ("element")) -> (w672:dbl[])
                  n148 = Build Array(2.0 ("element"), 0.0 ("element"), 0.0 ("element"), -30.0 ("element"), 1.0 ("element"), 0.9 ("element"), 0.6 ("element"), 1.0 ("element"), 1.0, 0.0 ("element")) -> (w671:dbl[])
                  n149 = Build Array(w674, w673, w672, w671) -> (w670:dbl[][])
                }
              }
            }
            frame True {
              # "ss"
              # "back away"
              # "turn at scale"
              n150 = global read "Robot Global Data.vi" "SweetSpot"() -> (w721:dbl)
              n151 = Build Array(4.0 ("element"), 0.45 ("element"), 140.0 ("element"), 0.0 ("element"), 0.0 ("element"), 0.0 ("element"), -0.3 ("element"), 0.0 ("element"), 0.0, 0.0 ("element")) -> (w715:dbl[])
              n152 = Build Array(3.0 ("element"), 0.4 ("element"), 0.0 ("element"), -90.0 ("element"), 0.0 ("element"), w721, -0.3 ("element"), 1.0 ("element"), 0.0, 1.0 ("element")) -> (w716:dbl[])
              n153 = Build Array(2.0 ("element"), 0.5 ("element"), 24.0 ("element"), -90.0 ("element"), 1.0 ("element"), w721, -0.3 ("element"), 1.0 ("element"), 1.0, 0.0 ("element")) -> (w717:dbl[])
              n154 = Build Array(3.0 ("element"), 0.0 ("element"), 0.0 ("element"), -90.0 ("element"), 1.0 ("element"), w721, 0.6 ("element"), 1.0 ("element"), 1.0, 0.0 ("element")) -> (w718:dbl[])
              n155 = Build Array(w715, w716, w717, w718) -> (w757:dbl[][])
            }
          }
          n156 = call "AutoArray.vi"("Array"=w650) -> ()
        }
        frame #2 {
          n157 = call "StopMotion.vi"() -> ()  [unwired: 12 in]
        }
      }
    }
    frame "RightSwitchOnly" {
      n158 = flat-sequence {
        frame #0 {
          n159 = call "StopMotion.vi"() -> ()  [unwired: 12 in]
          n160 = Wait (ms)(milliseconds to wait=u32 250) -> ()  [unwired: 1 out]
        }
        frame #1 {
          n161 = global read "Robot Global Data.vi" "Switch"() -> (w759:dbl)
          n162 = Greater?(x=w759, y=0.0) -> (0:w762:bool)
          n163 = case shown="True" w762 {
            tunnel: [w763 w775] -> w760
            frame False {
              # "2"
              n164 = Build Array(4.0 ("element"), 0.3 ("element"), 100.0 ("element"), 0.0 ("element"), 0.0 ("element"), 0.0 ("element"), 0.0 ("element"), 0.0 ("element"), 0.0 ("element"), 0.0 ("element")) -> (w764:dbl[])
              n165 = Build Array(w764) -> (w763:dbl[][])
            }
            frame True {
              # "ss"
              # "back away"
              # "turn at scale"
              n166 = global read "Robot Global Data.vi" "SweetSpot"() -> (w780:dbl)
              n167 = Build Array(4.0 ("element"), 0.45 ("element"), 140.0 ("element"), 0.0 ("element"), 0.0 ("element"), 0.0 ("element"), -0.3 ("element"), 0.0 ("element"), 0.0, 0.0 ("element")) -> (w779:dbl[])
              n168 = Build Array(3.0 ("element"), 0.4 ("element"), 0.0 ("element"), -90.0 ("element"), 0.0 ("element"), w780, -0.3 ("element"), 1.0 ("element"), 0.0, 1.0 ("element")) -> (w778:dbl[])
              n169 = Build Array(2.0 ("element"), 0.5 ("element"), 24.0 ("element"), -90.0 ("element"), 1.0 ("element"), w780, -0.3 ("element"), 1.0 ("element"), 1.0, 0.0 ("element")) -> (w777:dbl[])
              n170 = Build Array(2.0 ("element"), 0.0 ("element"), 0.0 ("element"), -90.0 ("element"), 1.0 ("element"), w780, 0.4 ("element"), 1.0 ("element"), 1.0, 0.0 ("element")) -> (w776:dbl[])
              n171 = Build Array(w779, w778, w777, w776) -> (w775:dbl[][])
            }
          }
          n172 = call "AutoArray.vi"("Array"=w760) -> ()
        }
        frame #2 {
          n173 = call "StopMotion.vi"() -> ()  [unwired: 12 in]
        }
      }
    }
    frame "Forward", Default {
      n174 = flat-sequence {
        frame #0 {
          n175 = call <vilib>:"Zero Yaw.vi"("Device Number"=FRIC_navX_DeviceNumbersTypeDef."Dev0", "Zero"=TRUE) -> ()  [unwired: 10 in]
        }
        frame #1 {
          n176 = call "StopMotion.vi"() -> ()  [unwired: 12 in]
          n177 = call <vilib>:"Zero Yaw.vi"("Device Number"=FRIC_navX_DeviceNumbersTypeDef."Dev0", "Zero"=TRUE) -> ()  [unwired: 10 in]
          n178 = Wait (ms)(milliseconds to wait=u32 500) -> ()  [unwired: 1 out]
        }
        frame #2 {
          # "2"
          n179 = Build Array(4.0 ("element"), 0.3 ("element"), 100.0 ("element"), 0.0 ("element"), 0.0 ("element"), 0.0 ("element"), 0.0 ("element"), 0.0 ("element"), 0.0 ("element"), 0.0 ("element")) -> (w825:dbl[])
          n180 = Build Array(w825) -> (w826:dbl[][])
          n181 = call "AutoArray.vi"("Array"=w826) -> ()
        }
        frame #3 {
          n182 = call "StopMotion.vi"() -> ()  [unwired: 12 in]
        }
      }
    }
    frame "Nothing" {
      n183 = call "StopMotion.vi"() -> ()  [unwired: 12 in]
    }
  }
